vi "Initialize Attributes.vi"(8 "error in (no error)":errorcluster, 10 "Attribute Data":variant, 11 "CS++Nanotec in":refnum<class "CS++Nanotec.lvclass">) -> (0 "error out":errorcluster, 2 "Found?":bool, 3 "CS++Nanotec out":refnum<class "CS++Nanotec.lvclass">)   [LabVIEW 2015, in "CS++Nanotec.lvlib" / "CS++Nanotec.lvclass"]
doc: "Initialize object attribute.\n\nUnique resources should be allocated elsewhere!"
uses:
  CS++Nanotec.lvclass
  CSPP_Core/Classes/CS++ProcessVariables/ProcessVariable/PV.lvclass
  CSPP_Core/Actors/CS++BaseActor/CS++BaseActor.lvclass/CS++BaseActor.ctl
  CSPP_Core/Actors/CS++DeviceActor/CS++DeviceActor.lvclass/CS++DeviceActor.ctl
  CSPP_Core/Classes/CS++ProcessVariables/ProcessVariable/PV.lvclass/PV.ctl
  CS++Nanotec.lvclass/CS++Nanotec.ctl
  CSPP_Core/Classes/CS++ProcessVariables/ProcessVariable/Write PV URL.vi
  CSPP_Core/Classes/CS++ProcessVariables/ProcessVariable/Write Type Descriptor.vi
  <vilib>/Utility/error.llb/Error Cluster From Error Code.vi
  CSPP_DeviceBase/CS++Motor/CS++Motor.lvclass
  CSPP_Core/Classes/CS++BaseClasses/Factory/CS++Factory.lvclass
  CSPP_Core/Libraries/Utilities/CS++Utilities.lvlib
  CSPP_Core/Classes/CS++ProcessVariables/CS++ProcessVariables.lvlib
  CSPP_Core/Actors/CS++BaseActor/CS++BaseActor.lvclass
  CSPP_Core/Actors/CS++DeviceActor/CS++DeviceActor.lvclass
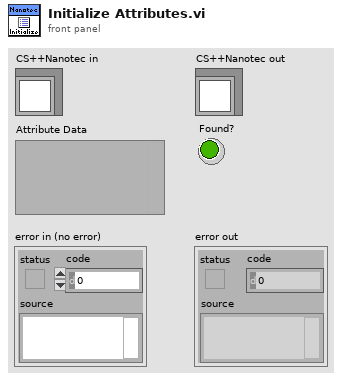
[diagram p1: front panel]
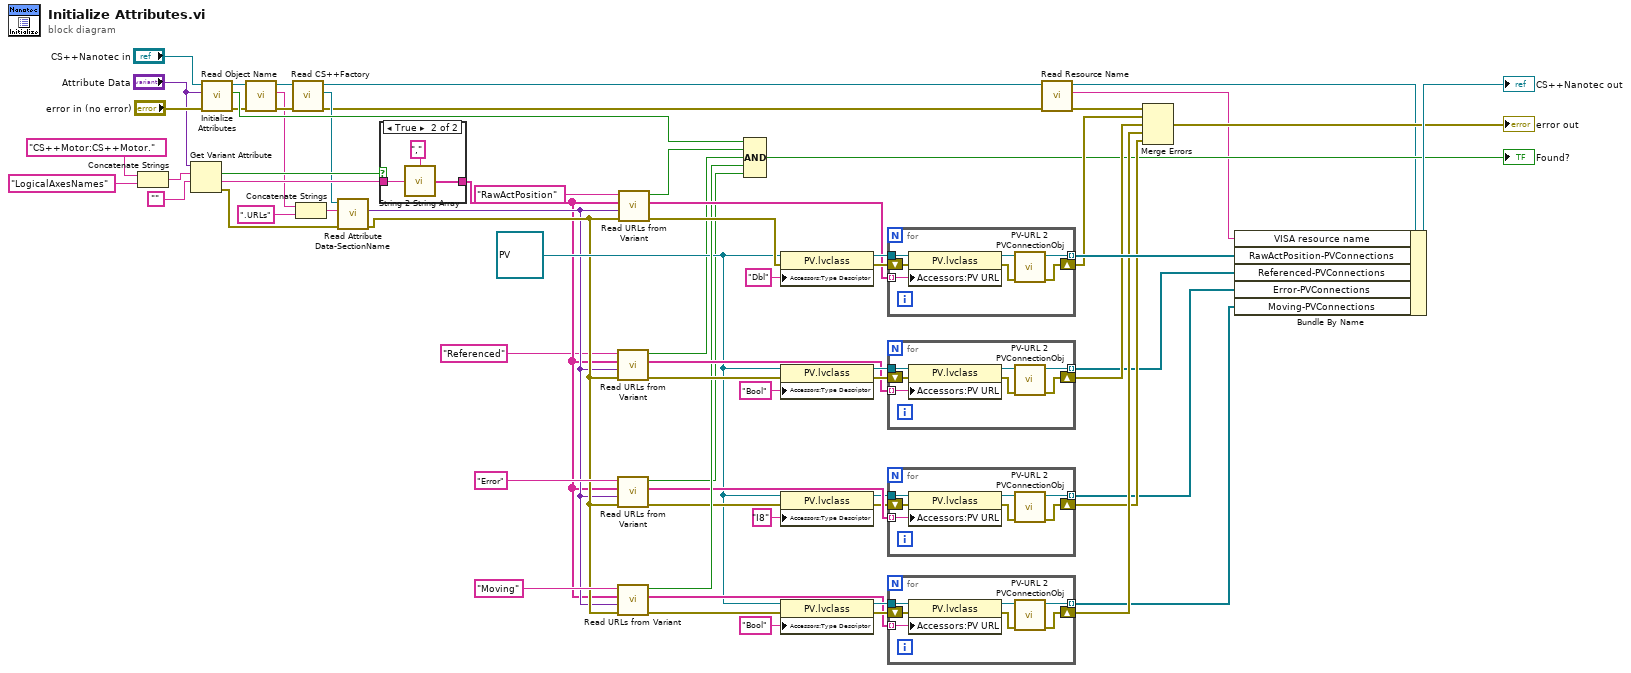
[diagram p0: block diagram]
diagram:
  w22 = refnum<class "PV.lvclass"> refnum ("CS++ProcessVariables.lvlib:PV.lvclass")
  n1 = Concatenate Strings("CS++Motor:CS++Motor.", "LogicalAxesNames" ("string")) -> (w65:string)
  n2 = Get Variant Attribute(Variant="Attribute Data", name=w65, default value (empty Variant)="") -> (found=w62:bool, value=w63:string, error out=w45:errorcluster)  [unwired: 1 in, 1 out]
  n3 = call-parent "Initialize Attributes.vi"("error in (no error)"="error in (no error)", "Attribute Data"="Attribute Data", "CS++Motor in"="CS++Nanotec in") -> ("error out"=w49:errorcluster, "Found?"=w50:bool, "CS++Motor out"=w48:refnum<class "CS++Nanotec.lvclass">)  [unwired: 6 in]
  n4 = call "Read Object Name.vi"("error in (no error)"=w49, "CS++BaseActor in"=w48) -> ("error out"=w51:errorcluster, "Object Name"=w43:string, "CS++BaseActor out"=w52:refnum<class "CS++Nanotec.lvclass">)  [unwired: 7 in]
  n5 = call "Read CS++Factory.vi"("error in (no error)"=w51, "CS++BaseActor in"=w52) -> ("error out"=w3:errorcluster, "CS++Factory"=w44:refnum<class "CS++Factory.lvclass">, "CS++BaseActor out"=w5:refnum<class "CS++Nanotec.lvclass">)  [unwired: 7 in]
  n6 = Concatenate Strings(w43, ".URLs" ("string")) -> (w47:string)
  n7 = call-dynamic "Read Attribute Data-SectionName.vi"("error in (no error)"=w45, "Object Name"=w47, "CS++Factory in"=w44) -> ("error out"=w20:errorcluster, "Attribute Data"=w19:variant)  [unwired: 6 in, 1 out]
  n8 = case shown="True" w62 {
    tunnel: w63 -> [_ w70]
    tunnel: [_ w69] -> w18
    frame False {
    }
    frame True {
      n9 = call "String 2 String Array.vi"("String"=w70, "Delimiter (\",\")"="," ("Delimiter (\",\")")) -> ("Substrings"=w69:string[])
    }
  }
  n10 = call "Read URLs from Variant.vi"("Error In"=w20, "URL Section Data"=w19, "Channel Names"=w18, "URL Prefix"="Referenced") -> ("Error Out"=w41:errorcluster, "URLs"=w38:string[], "Found?"=w15:bool)  [unwired: 4 in, 1 out]
  n11 = call "Read URLs from Variant.vi"("Error In"=w20, "URL Section Data"=w19, "Channel Names"=w18, "URL Prefix"="Error") -> ("Error Out"=w27:errorcluster, "URLs"=w26:string[], "Found?"=w21:bool)  [unwired: 4 in, 1 out]
  n12 = call "Read URLs from Variant.vi"("Error In"=w20, "URL Section Data"=w19, "Channel Names"=w18, "URL Prefix"="Moving") -> ("Error Out"=w32:errorcluster, "URLs"=w33:string[], "Found?"=w31:bool)  [unwired: 4 in, 1 out]
  n13 = call "Read URLs from Variant.vi"("Error In"=w20, "URL Section Data"=w19, "Channel Names"=w18, "URL Prefix"="RawActPosition") -> ("Error Out"=w56:errorcluster, "URLs"=w57:string[], "Found?"=w61:bool)  [unwired: 4 in, 1 out]
  n14 = Compound Arithmetic op=AND(w50, w61, w15, w31, w21) -> (→"Found?":bool)
  n15 = property class="PV.lvclass"(reference=w22, error in=w56, "Accessors:Type Descriptor"="Dbl" ("Type Descriptor")) -> (reference out=w59:refnum<class "PV.lvclass">, error out=w58:errorcluster)
  n16 = property class="PV.lvclass"(reference=w22, error in=w41, "Accessors:Type Descriptor"="Bool" ("Type Descriptor")) -> (reference out=w40:refnum<class "PV.lvclass">, error out=w39:errorcluster)
  n17 = property class="PV.lvclass"(reference=w22, error in=w27, "Accessors:Type Descriptor"="I8" ("Type Descriptor")) -> (reference out=w25:refnum<class "PV.lvclass">, error out=w24:errorcluster)
  n18 = property class="PV.lvclass"(reference=w22, error in=w32, "Accessors:Type Descriptor"="Bool" ("Type Descriptor")) -> (reference out=w34:refnum<class "PV.lvclass">, error out=w35:errorcluster)
  n19 = for {
    tunnel: w59 -> [w76]
    tunnel: w57 -> [w75] mode=indexing
    tunnel: [w74] -> w54 mode=indexing
    shift-right: [w73] -> w53
    shift-left: w58 -> [w71]
    n20 = property class="PV.lvclass"(reference=w76, error in=w71, "Accessors:PV URL"=w75) -> (reference out=w77:refnum<class "PV.lvclass">, error out=w72:errorcluster)
    n21 = call "PV-URL 2 PVConnectionObj.vi"("Error In"=w72, "PV"=w77) -> ("Error Out"=w73:errorcluster, "PVConnection"=w74:refnum<class "PVConnection.lvclass">)  [unwired: 7 in, 1 out]
  }
  n22 = for {
    tunnel: w40 -> [w83]
    tunnel: w38 -> [w82] mode=indexing
    tunnel: [w81] -> w13 mode=indexing
    shift-right: [w80] -> w37
    shift-left: w39 -> [w78]
    n23 = property class="PV.lvclass"(reference=w83, error in=w78, "Accessors:PV URL"=w82) -> (reference out=w84:refnum<class "PV.lvclass">, error out=w79:errorcluster)
    n24 = call "PV-URL 2 PVConnectionObj.vi"("Error In"=w79, "PV"=w84) -> ("Error Out"=w80:errorcluster, "PVConnection"=w81:refnum<class "PVConnection.lvclass">)  [unwired: 7 in, 1 out]
  }
  n25 = for {
    tunnel: w25 -> [w90]
    tunnel: w26 -> [w89] mode=indexing
    tunnel: [w88] -> w12 mode=indexing
    shift-right: [w87] -> w17
    shift-left: w24 -> [w85]
    n26 = property class="PV.lvclass"(reference=w90, error in=w85, "Accessors:PV URL"=w89) -> (reference out=w91:refnum<class "PV.lvclass">, error out=w86:errorcluster)
    n27 = call "PV-URL 2 PVConnectionObj.vi"("Error In"=w86, "PV"=w91) -> ("Error Out"=w87:errorcluster, "PVConnection"=w88:refnum<class "PVConnection.lvclass">)  [unwired: 7 in, 1 out]
  }
  n28 = for {
    tunnel: w34 -> [w97]
    tunnel: w33 -> [w96] mode=indexing
    tunnel: [w95] -> w14 mode=indexing
    shift-right: [w94] -> w29
    shift-left: w35 -> [w92]
    n29 = property class="PV.lvclass"(reference=w97, error in=w92, "Accessors:PV URL"=w96) -> (reference out=w98:refnum<class "PV.lvclass">, error out=w93:errorcluster)
    n30 = call "PV-URL 2 PVConnectionObj.vi"("Error In"=w93, "PV"=w98) -> ("Error Out"=w94:errorcluster, "PVConnection"=w95:refnum<class "PVConnection.lvclass">)  [unwired: 7 in, 1 out]
  }
  n31 = call "Read Resource Name.vi"("error in (no error)"=w3, "CS++DeviceActor in"=w5) -> ("error out"=w2:errorcluster, "Resource Name"=w1:string, "CS++DeviceActor out"=w4:refnum<class "CS++Nanotec.lvclass">)  [unwired: 7 in]
  n32 = Merge Errors(w2, w53, w37, w29, w17) -> (→"error out":errorcluster)
  n33 = Bundle By Name(cluster=w4, "VISA resource name"=w1, "RawActPosition-PVConnections"=w54, "Referenced-PVConnections"=w13, "Error-PVConnections"=w12, "Moving-PVConnections"=w14) -> (→"CS++Nanotec out":refnum<class "CS++Nanotec.lvclass">)
